vi "matrici_v0_v40.vi"() -> ()   [LabVIEW 2009]
uses:
  <vilib>/Math Plots/3D Math Plots/3D Surface/3D Surface XCtrl/3D Surface.xctl
  <vilib>/Math Plots/3D Math Plots/3D Surface/3D Surface Datatype/3D Surface Datatype.lvclass
  <vilib>/Math Plots/3D Math Plots/3D Surface/3D Surface Datatype/Public/Plot Helper (Vector).vi
  <vilib>/Analysis/Matrix/Numeric/Conversions/Array To Matrix - RA2.vi
  <vilib>/Analysis/Matrix/NI_Matrix.lvlib
panel:
  out "y":dbl=1.9999999999999982
  out "X":dbl=1.9999999999999982
  out "3D Surface":refnum<class "3D Plot Datatype.lvclass">[](xcontrol)
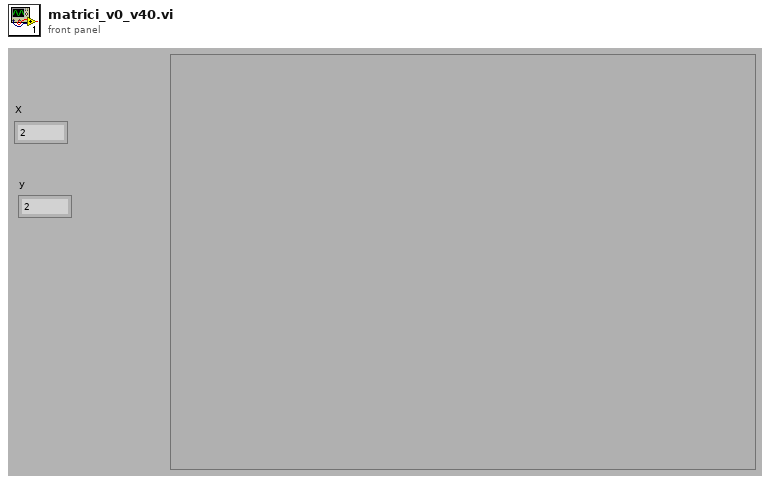
[diagram p1: front panel]
types:
  T1 = typedef "NI_Matrix.lvlib/RealMatrix.ctl" = dbl[][]
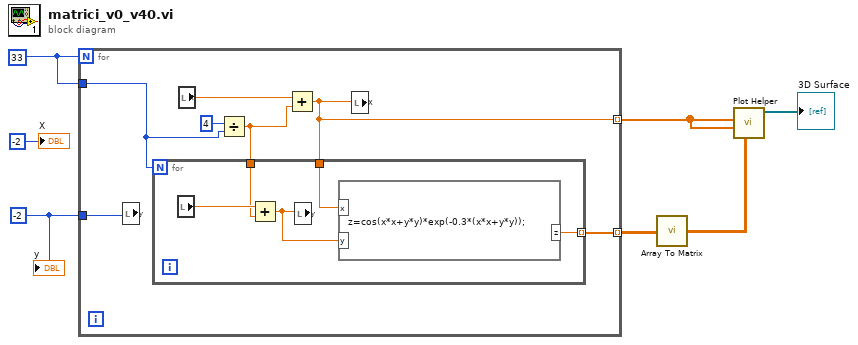
[diagram p0: block diagram]
diagram:
  w6 = 33
  w5 = -2
  n1 = for {
    N: w6 -> [_]
    tunnel: [w13] -> w1 mode=indexing
    tunnel: [w12] -> w4 mode=indexing
    tunnel: w6 -> [w10]
    tunnel: w5 -> [w8]
    n2 = local write "y"(w8) -> ()
    n3 = local read "X"() -> (w14:dbl)
    n4 = Divide(x=4, y=w10) -> (x/y=w9:dbl)
    n5 = Add(x=w14, y=w9) -> (x+y=w13:dbl)
    n6 = for {
      N: w10 -> [_]
      tunnel: w13 -> [w18]
      tunnel: [w16] -> w12 mode=indexing
      tunnel: w9 -> [w15]
      n7 = local read "y"() -> (w19:dbl)
      n8 = Add(x=w19, y=w15) -> (x+y=w17:dbl)
      n9 = local write "y"(w17) -> ()
      n10 = formula code="z=cos(x*x+y*y)*exp(-0.3*(x*x+y*y));"("x"=w18, "y"=w17) -> ("z"=w16:dbl)
    }
    n11 = local write "X"(w13) -> ()
  }
  n12 = call-poly <vilib>:"Array To Matrix.vi"("Real 2D Array"=w4) -> ("Real Matrix"=w2:T1)
  n13 = call-poly <vilib>:"Plot Helper.vi"("z matrix"=w2, "y vector"=w1, "x vector"=w1) -> ("3D Plot lvclass Array out"=→"3D Surface":refnum<class "3D Plot Datatype.lvclass">[])  [unwired: 3 in, 5 out]
  "X" <- -2
  "y" <- w5
